vi "RW All ECAT.vi"(2 "R/W Case":T30, 7 "RT Data in":T1={"Device ref"=0, "Scan Period (uSec)"=10000, "Device Channels"={"Status"={"BD Refs"=[], "Length"=0, "FIFO Index"=0, "Data"=[]}, "Command"={"BD Refs"=[], "Data"=[], "Length"=0, "FIFO Index"=0}}, "Local Chassis"=[], "EtherCAT Masters"=[], "Async"={"Status"=refnum, "Command"=refnum, "Input FIFO"=refnum, "Input FIFO buffer"=[], "Output FIFO"=refnum, "Output FIFO buffer"=[], "Async VI Ref"=refnum}, "ECAT Reconfig"={"Reconfig Module Found"=FALSE, "VI Ref"=refnum, "Status"=refnum}, "Device Error"={"status"=FALSE, "code"=0, "source"=""}, "DeviceName"="", "PCLSync?"=FALSE} {"Device Channels"."Status"."BD Refs"."Data Reference" format="%.0x"; "Device Channels"."Command"."BD Refs"."Data Reference" format="%.0x"; "Local Chassis"."FPGA"."VS ref" format="%.0x"; "Local Chassis"."RSI Modules"."VS ref" format="%.0x"; "Local Chassis"."VS ref" format="%.0x"; "Device ref" format="%.0x"; "EtherCAT Masters"."REM IO ECAT Slaves"."VS ref" format="%.0x"; "EtherCAT Masters"."Generic EtherCAT Slaves"."VS ref" format="%.0x"; "EtherCAT Masters"."VS ref" format="%.0x"; "EtherCAT Masters"."EtherCAT Slaves"."FPGA"."VS ref" format="%.0x"; "EtherCAT Masters"."EtherCAT Slaves"."RSI Modules"."VS ref" format="%.0x"; "EtherCAT Masters"."EtherCAT Slaves"."VS ref" format="%.0x"}) -> (8 "RT Data out":T1={"Device ref"=0, "Scan Period (uSec)"=10000, "Device Channels"={"Status"={"BD Refs"=[], "Length"=0, "FIFO Index"=0, "Data"=[]}, "Command"={"BD Refs"=[], "Data"=[], "Length"=0, "FIFO Index"=0}}, "Local Chassis"=[], "EtherCAT Masters"=[], "Async"={"Status"=refnum, "Command"=refnum, "Input FIFO"=refnum, "Input FIFO buffer"=[], "Output FIFO"=refnum, "Output FIFO buffer"=[], "Async VI Ref"=refnum}, "ECAT Reconfig"={"Reconfig Module Found"=FALSE, "VI Ref"=refnum, "Status"=refnum}, "Device Error"={"status"=FALSE, "code"=0, "source"=""}, "DeviceName"="", "PCLSync?"=FALSE} {"Device Channels"."Status"."BD Refs"."Data Reference" format="%.0x"; "Device Channels"."Command"."BD Refs"."Data Reference" format="%.0x"; "Local Chassis"."FPGA"."VS ref" format="%.0x"; "Local Chassis"."RSI Modules"."VS ref" format="%.0x"; "Local Chassis"."VS ref" format="%.0x"; "Device ref" format="%.0x"; "EtherCAT Masters"."REM IO ECAT Slaves"."VS ref" format="%.0x"; "EtherCAT Masters"."Generic EtherCAT Slaves"."VS ref" format="%.0x"; "EtherCAT Masters"."VS ref" format="%.0x"; "EtherCAT Masters"."EtherCAT Slaves"."FPGA"."VS ref" format="%.0x"; "EtherCAT Masters"."EtherCAT Slaves"."RSI Modules"."VS ref" format="%.0x"; "EtherCAT Masters"."EtherCAT Slaves"."VS ref" format="%.0x"})   [LabVIEW 2020, in "SEECD Engine.lvlib"]
uses:
  SEECD Engine.lvlib
  Type Defs/RW Case.ctl
  <vilib>/NI VeriStand/Custom Device API/Custom Device Item Ref.ctl
  <vilib>/NI VeriStand/Custom Device API/Custom Device API.lvlib
  <vilib>/NI VeriStand/Custom Device API/Data Reference.ctl
  <vilib>/NI VeriStand/Custom Device API/Block Data Reference.ctl
  Type Defs/Input Data.ctl
  Type Defs/Output Data.ctl
  Includes/Modules.lvlibp/RSI Module/Channel Type.ctl
  Includes/Modules.lvlibp/RSI Module/RSI Module.lvclass
  Includes/Modules.lvlibp/RSI Module/Module Models.ctl
  Type Defs/Module Config Data.ctl
  Type Defs/RSI Module Data.ctl
  Shared/Type Defs/UDV Data Type.ctl
  Shared/SEECD Shared.lvlib
  Shared/Type Defs/FXP Config.ctl
  Type Defs/UDV Data.ctl
  Type Defs/FPGA Data.ctl
  Type Defs/EtherCAT Slave Data.ctl
  Type Defs/EtherCAT Master Data.ctl
  Type Defs/Async Command.ctl
  Type Defs/Async State.ctl
  Type Defs/Async Status.ctl
  Type Defs/Async Data.ctl
  Type Defs/Mixed IO.ctl
  Type Defs/Local Chassis Data.ctl
  Type Defs/ECAT Reconfig State.ctl
  Type Defs/ECAT Reconfig Status.ctl
  Type Defs/ECAT Reconfig Data.ctl
  Type Defs/Device Channels.ctl
  Type Defs/RT Data.ctl
  Type Defs/Open Module IOVs.ctl
  Type Defs/Mod Size Indexes.ctl
  Type Defs/Generic ECAT Slave IOV Cluster.ctl
  Type Defs/Generic ECAT Slave Data Cluster.ctl
  Type Defs/Generic ECAT Slave RT-Data-Array.ctl
  Type Defs/REM IO ECAT Slave IOV Cluster.ctl
  Type Defs/REM IO ECAT Slave Data Cluster.ctl
  Type Defs/REM IO ECAT Slave RT-Data-Array.ctl
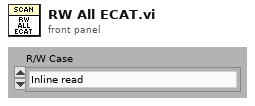
[diagram p1: front panel]
types:
  T1 = typedef "SEECD Engine.lvlib/RT Data.ctl" = cluster{"Device ref":T2, "Scan Period (uSec)":u32, "Device Channels":T3, "Local Chassis":T8[], "EtherCAT Masters":T20[], "Async":T28, "ECAT Reconfig":T29, "Device Error":errorcluster, "DeviceName":string, "PCLSync?":bool}
  T2 = typedef "Custom Device API.lvlib/Custom Device Item Ref.ctl" = u64
  T3 = typedef "SEECD Engine.lvlib/Device Channels.ctl" = cluster{"Status":T4, "Command":T7}
  T4 = typedef "SEECD Engine.lvlib/Output Data.ctl" = cluster{"BD Refs":T5[], "Length":i32, "FIFO Index":i32, "Data":dbl[]}
  T5 = typedef "Custom Device API.lvlib/Block Data Reference.ctl" = cluster{"Data Reference":T6, "Offset":u64, "Length":u64}
  T6 = typedef "Custom Device API.lvlib/Data Reference.ctl" = i32
  T7 = typedef "SEECD Engine.lvlib/Input Data.ctl" = cluster{"BD Refs":T5[], "Data":dbl[], "Length":i32, "FIFO Index":i32}
  T8 = typedef "SEECD Engine.lvlib/Local Chassis Data.ctl" = cluster{"VS ref":T2, "RSI Modules":T9[], "FPGA":T15[], "Input Mod Size Idxs":T19, "Output Modules":i32[], "MixedIO Mod Size Idxs":T19}
  T9 = typedef "SEECD Engine.lvlib/RSI Module Data.ctl" = cluster{"VS ref":T2, "IOV ref":refnum<k21>, "Open Mod refs":T10, "Module DVR":refnum<data-value>, "Slot":u32, "Model":T11, "Channel Type":T12, "EtherCAT?":bool, "CDInput Data":T7, "CDOutput Data":T4, "Module Config Data":T13, "Mixed IO":T14}
  T10 = typedef "SEECD Engine.lvlib/Open Module IOVs.ctl" = cluster{"Analog Read":refnum<k21>, "Digital Read":refnum<k21>, "Analog Write":refnum<k21>, "Digital Write":refnum<k21>}
  T11 = typedef "Modules.lvlibp/RSI Module.lvclass/Module Models.ctl" = enum16{"Empty", "NI 9201", "NI 9203", "NI 9205", "NI 9206", "NI 9207", "NI 9208", "NI 9209", "NI 9210", "NI 9211", "NI 9212", "NI 9213", "NI 9214", "NI 9215", "NI 9216", "NI 9217", "NI 9219", "NI 9220", "NI 9221", "NI 9222", "NI 9223", "NI 9224", "NI 9225", "NI 9226", "NI 9227", "NI 9228", "NI 9229", "NI 9233", "NI 9234", "NI 9235", "NI 9236", "NI 9237", "NI 9239", "NI 9242", "NI 9244", "NI 9253", "NI 9263", "NI 9264", "NI 9265", "NI 9266", "NI 9269", "NI 9344", "NI 9350", "NI 9375", "NI 9401", "NI 9402", "NI 9403", "NI 9411", "NI 9421", "NI 9422", "NI 9423", "NI 9425", "NI 9426", "NI 9435", "NI 9436", "NI 9437", "NI 9472", "NI 9474", "NI 9475", "NI 9476", "NI 9477", "NI 9478", "NI 9481", "NI 9482", "NI 9485"}
  T12 = typedef "Modules.lvlibp/RSI Module.lvclass/Channel Type.ctl" = enum16{"Analog", "Digital"}
  T13 = typedef "SEECD Engine.lvlib/Module Config Data.ctl" = cluster{"Configurable?":bool, "Config Block Data Refs":T5[], "Config Data DVR":refnum<data-value>, "Previous Values":dbl[], "Local Reconfig VI Ref":refnum<vi>}
  T14 = typedef "SEECD Engine.lvlib/Mixed IO.ctl" = cluster{"Input Channel Indices":i32[], "Input Buffer":dbl[]}
  T15 = typedef "SEECD Engine.lvlib/FPGA Data.ctl" = cluster{"VS ref":T2, "IOV ref":refnum<k21>, "FPGA Target":enum16{"Local", "EtherCAT"}, "Product Code":u32, "Bitfile Signature":string, "Bitfile Path (RT)":path, "FPGA Session":u32, "Input Data":T7, "Output Data":T4, "UDVs":cluster{"From FPGA":T16[], "To FPGA":T16[]}}
  T16 = typedef "SEECD Engine.lvlib/UDV Data.ctl" = cluster{"VS ref":T2, "IOV Ref":refnum<k21>, "Name":string, "UDV Data Type":T17, "Supported Type?":bool, "FXP Config":T18, "FXP VI Ref":refnum<vi>}
  T17 = typedef "SEECD Shared.lvlib/UDV Data Type.ctl" = enum16{"Boolean", "Fixed Point", "Int8", "Int16", "Int32", "Int64", "U32 Bit Field", "UInt8", "UInt16", "UInt32", "UInt64", "Other", "DBL", "SGL"}
  T18 = typedef "SEECD Shared.lvlib/FXP Config.ctl" = cluster{"signed":bool, "size":u32, "integersize":i32}
  T19 = typedef "SEECD Engine.lvlib/Mod Size Indexes.ctl" = cluster{"4":i32[], "8":i32[], "16":i32[], "32":i32[], "other":i32[]}
  T20 = typedef "SEECD Engine.lvlib/EtherCAT Master Data.ctl" = cluster{"VS ref":T2, "IOV ref":refnum<k21>, "Master ID":u32, "Cyclic Data Bandwidth":u32, "EtherCAT Slaves":T21[], "Generic EtherCAT Slaves":T22, "REM IO ECAT Slaves":T25}
  T21 = typedef "SEECD Engine.lvlib/EtherCAT Slave Data.ctl" = cluster{"VS ref":T2, "IOV ref":refnum<k21>, "Position Address":u16, "RSI Modules":T9[], "FPGA":T15[], "Input Mod Size Idxs":T19, "Output Modules":i32[], "MixedIO Mod Size Idxs":T19}
  T22 = typedef "SEECD Engine.lvlib/Generic ECAT Slave RT-Data-Array.ctl" = T23[]
  T23 = typedef "SEECD Engine.lvlib/Generic ECAT Slave Data Cluster.ctl" = cluster{"VS ref":T2, "IOV ref":refnum<k21>, "Position Address":u16, "I/O Imput Vars ":T24[], "I/O Output Vars":T24[], "I/O Input Data":T7, "I/O Output Data":T4, "Distributed Clock":bool}
  T24 = typedef "SEECD Engine.lvlib/Generic ECAT Slave IOV Cluster.ctl" = cluster{"VS ref":T2, "IOV Ref":refnum<k21>, "Name":string, "UDV Data Type":T17}
  T25 = typedef "SEECD Engine.lvlib/REM IO ECAT Slave RT-Data-Array.ctl" = T26[]
  T26 = typedef "SEECD Engine.lvlib/REM IO ECAT Slave Data Cluster.ctl" = cluster{"VS ref":T2, "IOV ref":refnum<k21>, "Position Address":u16, "I/O Imput Vars ":T27[], "I/O Output Vars":T27[], "I/O Input Data":T7, "I/O Output Data":T4}
  T27 = typedef "SEECD Engine.lvlib/REM IO ECAT Slave IOV Cluster.ctl" = cluster{"VS ref":T2, "IOV Ref":refnum<k21>, "Name":string, "UDV Data Type":T17, "Scaling Factor":dbl}
  T28 = typedef "SEECD Engine.lvlib/Async Data.ctl" = cluster{"Status":refnum<queue>, "Command":refnum<queue>, "Input FIFO":refnum<k33>, "Input FIFO buffer":dbl[], "Output FIFO":refnum<k33>, "Output FIFO buffer":dbl[], "Async VI Ref":refnum<vi>}
  T29 = typedef "SEECD Engine.lvlib/ECAT Reconfig Data.ctl" = cluster{"Reconfig Module Found":bool, "VI Ref":refnum<vi>, "Status":refnum<queue>}
  T30 = typedef "SEECD Engine.lvlib/RW Case.ctl" = enum16{"Inline read", "Inline write", "Async - Inline loop read", "Async - Inline loop write", "Async loop (read/write)"}
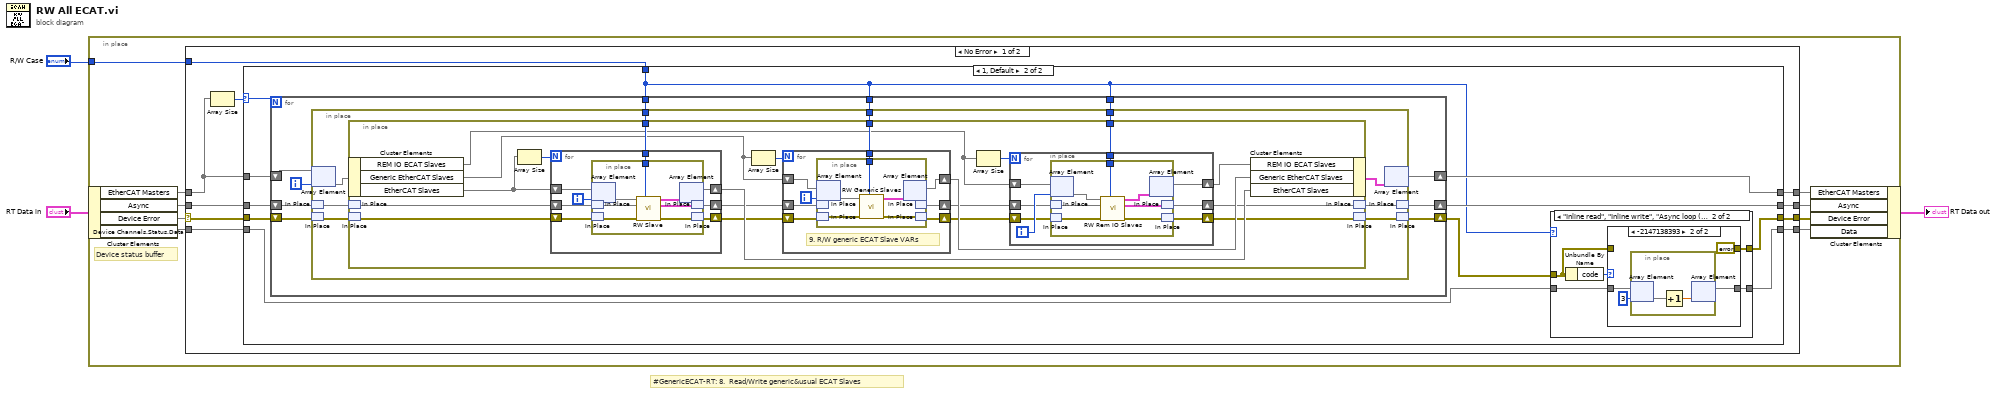
[diagram p0: block diagram]
diagram:
  # "#GenericECAT-RT: 8.  Read/Write generic&usual ECAT Slaves"
  n1 = in-place {
    in-place-border: "R/W Case" -> [w6]
    # "Device status buffer"
    n2 = in-place-cluster #1("RT Data in") -> ("EtherCAT Masters"=w7, "Async"=w9, "Device Error"=w12, "Device Channels.Status.Data"=w5)
    n3 = case shown="No Error" w12 {
      selector: w12 -> [w20 w140]
      tunnel: [w15 w140] -> w11
      tunnel: [w18 w139] -> w10
      tunnel: w9 -> [w21 w139]
      tunnel: [w19 w138] -> w8
      tunnel: w7 -> [w22 w138]
      tunnel: w6 -> [w17 _]
      tunnel: w5 -> [w16 w137]
      tunnel: [w13 w137] -> w4
      frame No Error {
        n4 = Array Size(array=w22) -> (size(s)=w14:i32)
        n5 = case shown="1, Default" w14 {
          selector: w14 -> [_ w30]
          tunnel: w22 -> [w26 w28]
          tunnel: w21 -> [w25 w31]
          tunnel: w20 -> [w24 w37]
          tunnel: [w26 w32] -> w19
          tunnel: [w25 w29] -> w18
          tunnel: w17 -> [_ w27]
          tunnel: w16 -> [w23 w34]
          tunnel: [w24 w35] -> w15
          tunnel: [w23 w33] -> w13
          frame 0 {
          }
          frame 1, Default {
            n6 = for {
              N: w30 -> [_]
              shift-right: [w56] -> w36
              shift-left: w37 -> [w57]
              shift-right: [w60] -> w32
              shift-left: w28 -> [w62]
              shift-right: [w58] -> w29
              shift-left: w31 -> [w59]
              tunnel: w27 -> [w55]
              tunnel: w27 -> [w54]
              tunnel: w27 -> [w53]
              i -> [w61]
              n7 = in-place {
                in-place-border: w55 -> [w65]
                in-place-border: w54 -> [w64]
                in-place-border: w53 -> [w63]
                n8 = in-place-array #2(w62, w61) -> (w71)
                n9 = in-place-match #3(w59) -> (w69)
                n10 = in-place-match #4(w57) -> (w67:errorcluster)
                n11 = in-place {
                  in-place-border: w65 -> [w88]
                  in-place-border: w64 -> [w83]
                  in-place-border: w63 -> [w77]
                  n12 = in-place-cluster #5(w71) -> ("REM IO ECAT Slaves"=w72, "Generic EtherCAT Slaves"=w82, "EtherCAT Slaves"=w87)
                  n13 = in-place-match #6(w69) -> (w90)
                  n14 = in-place-match #7(w67) -> (w89:errorcluster)
                  n15 = Array Size(array=w87) -> (size(s)=w91:i32)
                  n16 = for {
                    N: w91 -> [_]
                    shift-right: [w127] -> w86
                    shift-left: w87 -> [w129]
                    shift-right: [w122] -> w84
                    shift-left: w89 -> [w123]
                    shift-right: [w125] -> w85
                    shift-left: w90 -> [w126]
                    tunnel: w88 -> [w124]
                    i -> [w128]
                    n17 = in-place {
                      in-place-border: w124 -> [w131]
                      n18 = in-place-array #8(w129, w128) -> (w130)
                      n19 = in-place-match #9(w126) -> (w132)
                      n20 = in-place-match #10(w123) -> (w134:errorcluster)
                      n21 = call "RW Slave.vi"("R/W Case"=w131, "error in (no error)"=w134, "Async in"=w132, "Slave in"=w130) -> ("error out"=w133:errorcluster, "Async out"=w135:T28, "Slave out"=w136:T21)  [unwired: 5 in]
                      n22 = in-place-array #8(w136) -> (w127)  [unwired: 1 out]
                      n23 = in-place-match #9(w135) -> (w125)
                      n24 = in-place-match #10(w133) -> (w122:errorcluster)
                    }
                  }
                  n25 = Array Size(array=w82) -> (size(s)=w81:i32)
                  n26 = for {
                    N: w81 -> [_]
                    shift-right: [w110] -> w78
                    shift-left: w84 -> [w111]
                    shift-right: [w109] -> w79
                    shift-left: w85 -> [w112]
                    shift-right: [w113] -> w80
                    shift-left: w82 -> [w114]
                    tunnel: w83 -> [w108]
                    i -> [w107]
                    # "9. R/W generic ECAT Slave VARs"
                    n27 = in-place {
                      in-place-border: w108 -> [w119]
                      n28 = in-place-array #11(w114, w107) -> (w121)
                      n29 = in-place-match #12(w112) -> (w116)
                      n30 = in-place-match #13(w111) -> (w118:errorcluster)
                      n31 = call "RW Generic Slaves.vi"("R/W Case"=w119, "error in (no error)"=w118, "Async in"=w116, "Generic ECAT Slaves in"=w121) -> ("error out"=w117:errorcluster, "Async out"=w115:T28, "Generic ECAT Slaves out"=w120:T23)  [unwired: 5 in]
                      n32 = in-place-array #11(w120) -> (w113)  [unwired: 1 out]
                      n33 = in-place-match #12(w115) -> (w109)
                      n34 = in-place-match #13(w117) -> (w110:errorcluster)
                    }
                  }
                  n35 = Array Size(array=w72) -> (size(s)=w73:i32)
                  n36 = for {
                    N: w73 -> [_]
                    shift-right: [w93] -> w76
                    shift-left: w72 -> [w99]
                    shift-right: [w95] -> w75
                    shift-left: w79 -> [w97]
                    shift-right: [w94] -> w74
                    shift-left: w78 -> [w96]
                    tunnel: w77 -> [w92]
                    i -> [w98]
                    n37 = in-place {
                      in-place-border: w92 -> [w100]
                      n38 = in-place-array #14(w99, w98) -> (w102)
                      n39 = in-place-match #15(w97) -> (w105)
                      n40 = in-place-match #16(w96) -> (w106:errorcluster)
                      n41 = call "RW Rem IO Slaves.vi"("R/W Case"=w100, "error in (no error)"=w106, "Async in"=w105, "REM IO EtherCAT Slave In"=w102) -> ("error out"=w104:errorcluster, "Async out"=w103:T28, "REM IO EtherCAT Slave Out"=w101:T26)  [unwired: 5 in]
                      n42 = in-place-array #14(w101) -> (w93)  [unwired: 1 out]
                      n43 = in-place-match #15(w103) -> (w95)
                      n44 = in-place-match #16(w104) -> (w94:errorcluster)
                    }
                  }
                  n45 = in-place-cluster #5("REM IO ECAT Slaves"=w76, "Generic EtherCAT Slaves"=w80, "EtherCAT Slaves"=w86) -> (w70:cluster{})
                  n46 = in-place-match #6(w75) -> (w68)
                  n47 = in-place-match #7(w74) -> (w66:errorcluster)
                }
                n48 = in-place-array #2(w70) -> (w60)  [unwired: 1 out]
                n49 = in-place-match #3(w68) -> (w58)
                n50 = in-place-match #4(w66) -> (w56:errorcluster)
              }
            }
            n51 = case shown="\"Inline read\", \"Inline write\", \"Async loop (read/write)\"" w27 {
              tunnel: w36 -> [w39 w43]
              tunnel: [w39 w42] -> w35
              tunnel: w34 -> [w38 w41]
              tunnel: [w38 w40] -> w33
              frame Default {
              }
              frame "Inline read", "Inline write", "Async loop (read/write)" {
                n52 = Unbundle By Name(w43) -> ("code"=w44:i32)
                n53 = case shown="-2147138393" w44 {
                  tunnel: w43 -> [w46 _]
                  tunnel: [w46 errorcluster {"status"=FALSE, "code"=0, "source"=""} ("error IO")] -> w42
                  tunnel: [w45 w47] -> w40
                  tunnel: w41 -> [w45 w49]
                  frame 0, Default {
                  }
                  frame -2147138393 {
                    n54 = in-place {
                      n55 = in-place-array #17(w49, 3) -> (w52)
                      n56 = Increment(x=w52) -> (x+1=w51:dbl)
                      n57 = in-place-array #17(w51) -> (w47)  [unwired: 1 out]
                    }
                  }
                }
              }
            }
          }
        }
      }
      frame Error {
      }
    }
    n58 = in-place-cluster #1("EtherCAT Masters"=w8, "Async"=w10, "Device Error"=w11, "Data"=w4) -> (→"RT Data out":cluster{})
  }
